vi "Read N Bytes.vi"(0 "COM Port":refnum<visa-resource-name>, 1 "NFC ID(ASCII)":string, 5 "Sector":i32 format="%x", 7 "Starting Page Address":i32 format="%x", 9 "Offset(0-3, Byte)":i32 max=16 step=1, 11 "Length(Byte)":i32, 12 "Reverse Output[F]":bool) -> (4 "PN532 COM Port out":refnum<visa-resource-name>, 6 "Data(Hex)":string, 8 "Data(ASCII)":string, 15 "error out":errorcluster)   [LabVIEW 2012, in "NFC Driver.lvlib"]
uses:
  NFC Driver.lvlib
  <vilib>/Utility/error.llb/Error Cluster From Error Code.vi
  <vilib>/ErrorRing/Error Ring.xnode
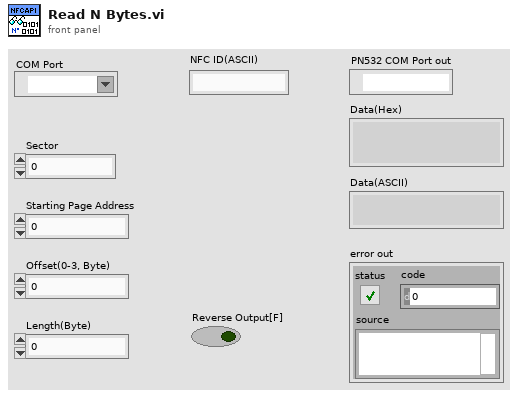
[diagram p1: front panel]
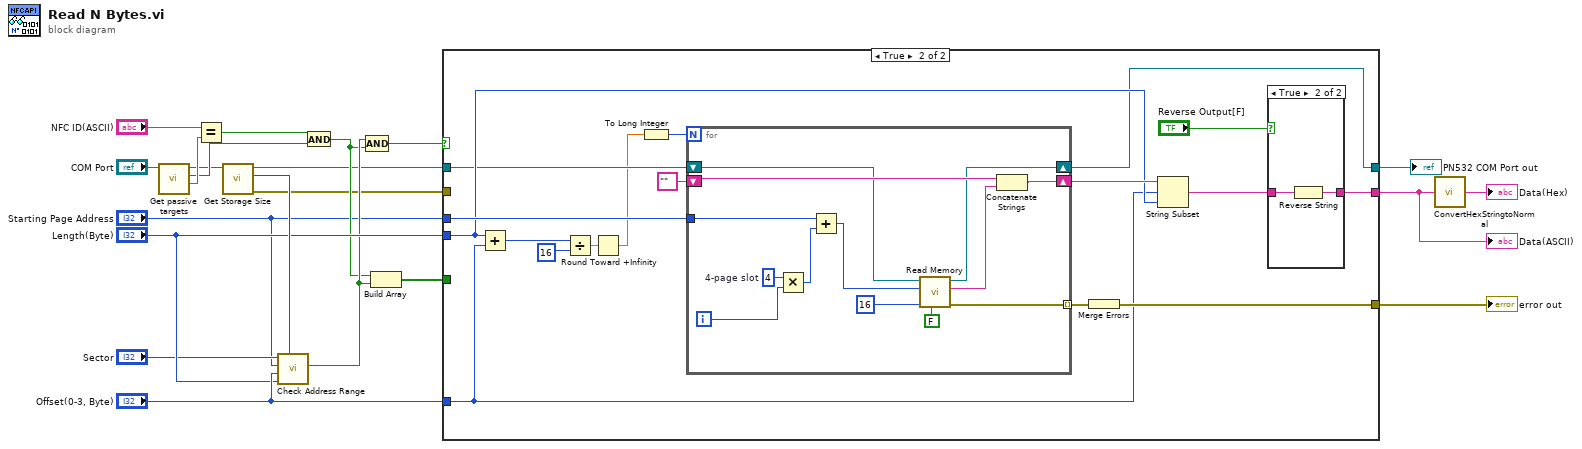
[diagram p0: block diagram]
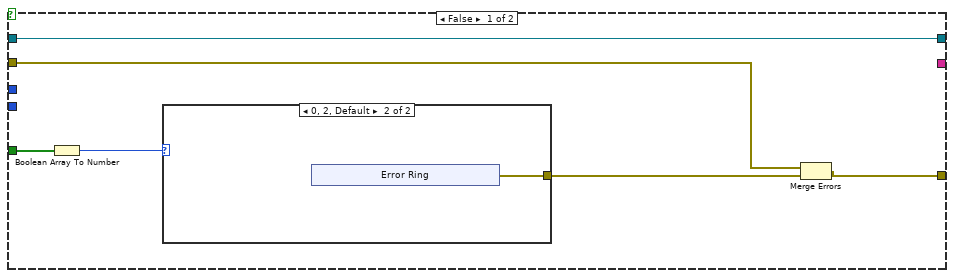
[diagram p2: hidden frame]
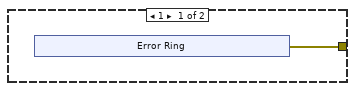
[diagram p3: hidden frame]
diagram:
  n1 = call "Get passive targets.vi"("PN532 COM Port"="COM Port") -> ("NFC ID (ASCII)"=w19:string, "Found?"=w11:bool, "PN532 COM Port Out"=w4:refnum<visa-resource-name>)  [unwired: 6 in, 2 out]
  n2 = Equal?(x="NFC ID(ASCII)", y=w19) -> (x = y?=w12:bool)
  n3 = call "Get Storage Size.vi"("PN532 COM Port"=w4) -> ("error out"=w2:errorcluster, "Storage Size"=w18:i32, "PN532 COM Port out"=w3:refnum<visa-resource-name>)  [unwired: 8 in]
  n4 = call "Check Address Range.vi"("Storage Size"=w18, "Length(Byte)"="Length(Byte)", "Offset"="Offset(0-3, Byte)", "Page(hex)"="Starting Page Address", "Sector"="Sector") -> ("Address In Range"=w14:bool)  [unwired: 6 in]
  n5 = And(x=w12, y=w11) -> (x .and. y?=w10:bool)
  n6 = Compound Arithmetic op=AND(w14, w10) -> (w15:bool)
  n7 = Build Array(w10, w14) -> (w13:bool[])
  n8 = case shown="True" w15 {
    tunnel: "Starting Page Address" -> [_ w56]
    tunnel: [w25 w54] -> w21
    tunnel: "Length(Byte)" -> [_ w52]
    tunnel: "Offset(0-3, Byte)" -> [_ w51]
    tunnel: [_ w49] -> w7
    tunnel: w3 -> [w22 w47]
    tunnel: w2 -> [w27 _]
    tunnel: w13 -> [w24 _]
    tunnel: [w22 w40] -> w1
    frame False {
      n9 = Boolean Array To Number(Boolean array=w24) -> (number=w23:u32)
      n10 = case shown="0, 2, Default" w23 {
        tunnel: [w28 w34] -> w26
        frame 1 {
          n11 = xnode "Error Ring"() -> ("error out"=w28:errorcluster)
        }
        frame 0, 2, Default {
          n12 = xnode "Error Ring"() -> ("error out"=w34:errorcluster)
        }
      }
      n13 = Merge Errors(w27, w26) -> (w25:errorcluster)
    }
    frame True {
      n14 = Add(x=w52, y=w51) -> (x+y=w53:i32)
      n15 = Divide(x=w53, y=u16 16) -> (x/y=w42:dbl)
      n16 = Round Toward +Infinity(x=w42) -> (ceil(x): smallest int >= x=w41:dbl)
      n17 = To Long Integer(number=w41) -> (32bit integer=w46:i32)
      n18 = for {
        N: w46 -> [_]
        shift-right: [w57] -> w40
        shift-left: w47 -> [w58]
        tunnel: [w67] -> w45 mode=indexing
        shift-right: [w66] -> w55
        shift-left: "" ("16-byte data") -> [w65]
        tunnel: w56 -> [w69]
        i -> [w63]
        w62 = 4  # 4-page slot
        n19 = Multiply(x=w62, y=w63) -> (x*y=w61:i32)
        n20 = Add(x=w69, y=w61) -> (x+y=w68:i32)
        n21 = call "Read Memory.vi"("Reverse Output[F]"=FALSE ("Reverse Output"), "length (Byte, max. 16)"=16 ("length (max. 16)"), "Page Address"=w68, "PN532 COM Port"=w58) -> ("error out"=w67:errorcluster, "16-byte data(Hex)"=w59:string, "PN532 COM Port Out"=w57:refnum<visa-resource-name>)  [unwired: 3 in, 2 out]
        n22 = Concatenate Strings(w65, w59) -> (w66:string)
      }
      n23 = Merge Errors(w45) -> (w54:errorcluster)
      n24 = String Subset(string=w55, offset (0)=w51, length (rest)=w52) -> (substring=w50:string)
      n25 = case shown="True" "Reverse Output[F]" {
        tunnel: [w70 w71] -> w49
        tunnel: w50 -> [w70 w72]
        frame False {
        }
        frame True {
          n26 = Reverse String(1:w72) -> (0:w71:string)
        }
      }
    }
  }
  "error out" <- w21
  "Data(ASCII)" <- w7
  "PN532 COM Port out" <- w1
  n27 = call "ConvertHexStringtoNormal.vi"("Hex String"=w7) -> ("Normal String"=→"Data(Hex)":string)
